vi "EAGLE GUI V5.vi"(9 "TableIn":string[][](table)) -> ()   [LabVIEW 2015]
uses:
  Stream/Controls/RT Status Refs.ctl
  Stream/Robo Team Engine Command.ctl
  Stream/Robo Team Globals.vi
panel:
  out "ViewFinder Sign":picture
  out "Frame Rec":u32
  out "AlgoTime":u32
  out "FrameRate":dbl format="%#.1f"
  out "Stopped":bool
  out "Table Control":string[][](table)
  in  "Ranging":u32
  in  "Aiming":u32
  in  "Illume":u32
  in  "close":bool
  in  "Previous":bool
  in  "Next":bool
  in  "RangingIntensity":u32(slide)=1 caption="Ranging\nIntensity" max=10 step=1 scale=0.0..10.0
  in  "AimingIntensity":u32(slide)=1 caption="Aiming\nIntensity" max=10 step=1 scale=0.0..10.0
  in  "IlluminationIntensity":u32(slide)=1 caption="Illumination\nIntensity" max=10 step=1 scale=0.0..10.0
  out "Iris Found Status":bool
  in  "Tab":enum32{"Page 1", "Page 2", "Page 3"}(tab)
  out "Image":T1(plugin-control)
  # "Treatment Info"
  # "Treatment Process"
  # "Illumination Settings"
  # "Instructions"
  # "1. Adjust illumination\n2. Align the green cross to \n    the center of the pupil\n3. Form cross from the two\n    red lines (Ranging Beams)"
  # "Instructions"
  # "Limbus Border Found\nReady\nClick START"
  # "Instructions"
  # "READY!\n\nClick Start"
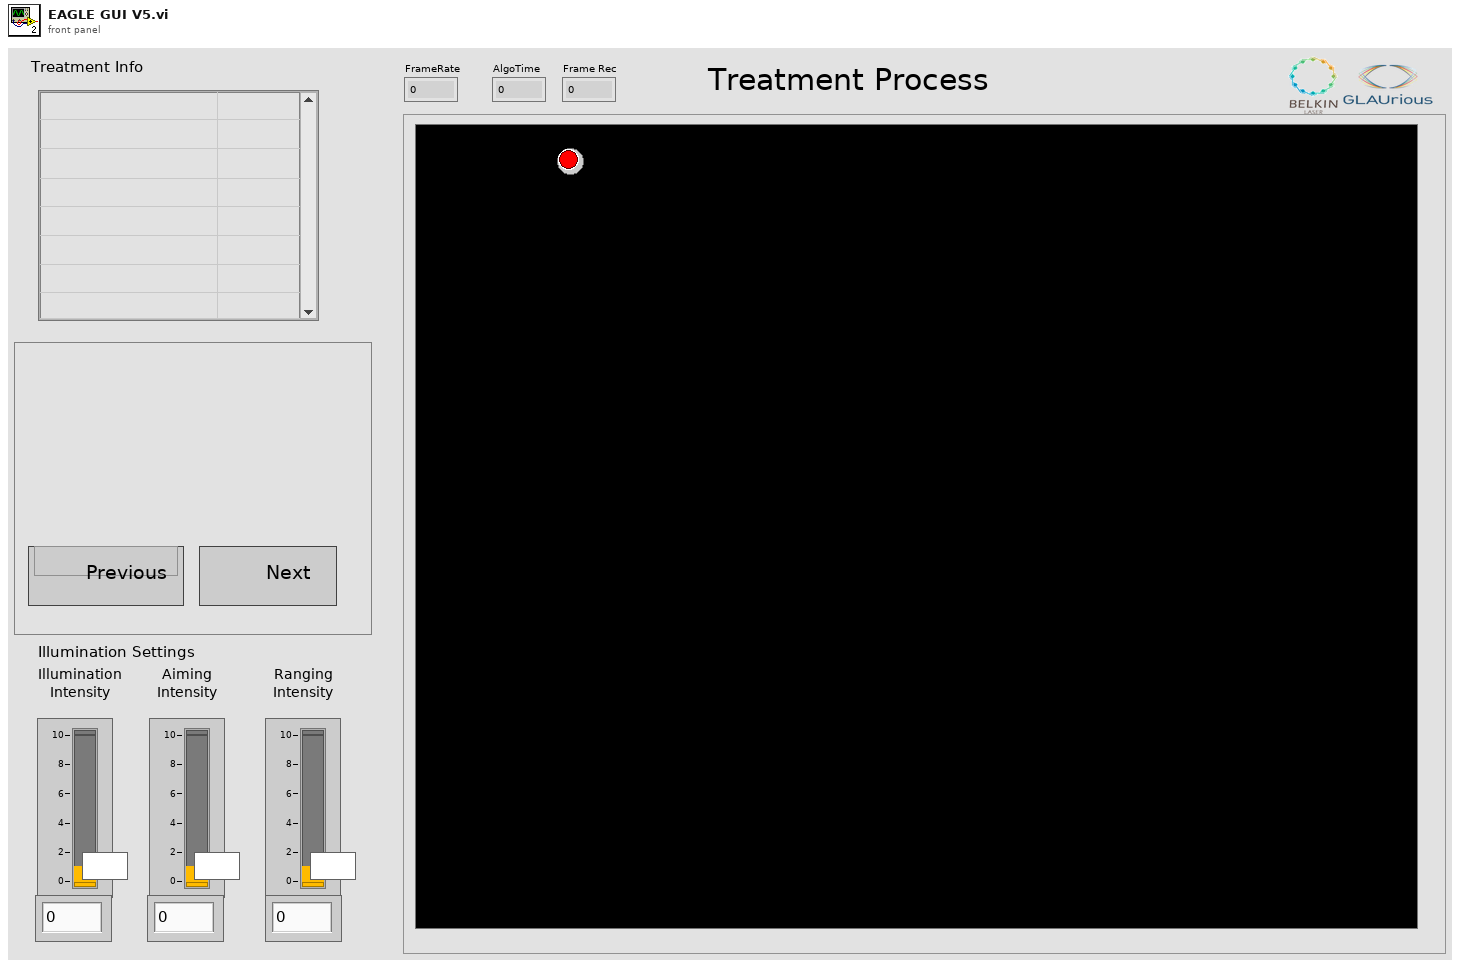
[diagram p1: front panel]
types:
  T1 = typedef "IMAQ Image.ctl" = refnum<image>
  T2 = typedef "RT Status Refs.ctl" = cluster{"Algo Time ref":refnum<vi>, "FrameRate ref":refnum<vi>, "FrameRecRef":refnum<vi>}
  T3 = typedef "Robo Team Engine Command.ctl" = cluster{"Command":string, "Data":variant, "Error":errorcluster, "Timeout":i32}
  T4 = enum8{"Enabled", "Disabled", "Disabled and Grayed Out"}
  T5 = typedef "LVPositionTypeDef.ctl" = cluster{"Left":i32, "Top":i32}
  T6 = typedef "LVRectTypeDef.ctl" = cluster{"Left":i16, "Top":i16, "Right":i16, "Bottom":i16}
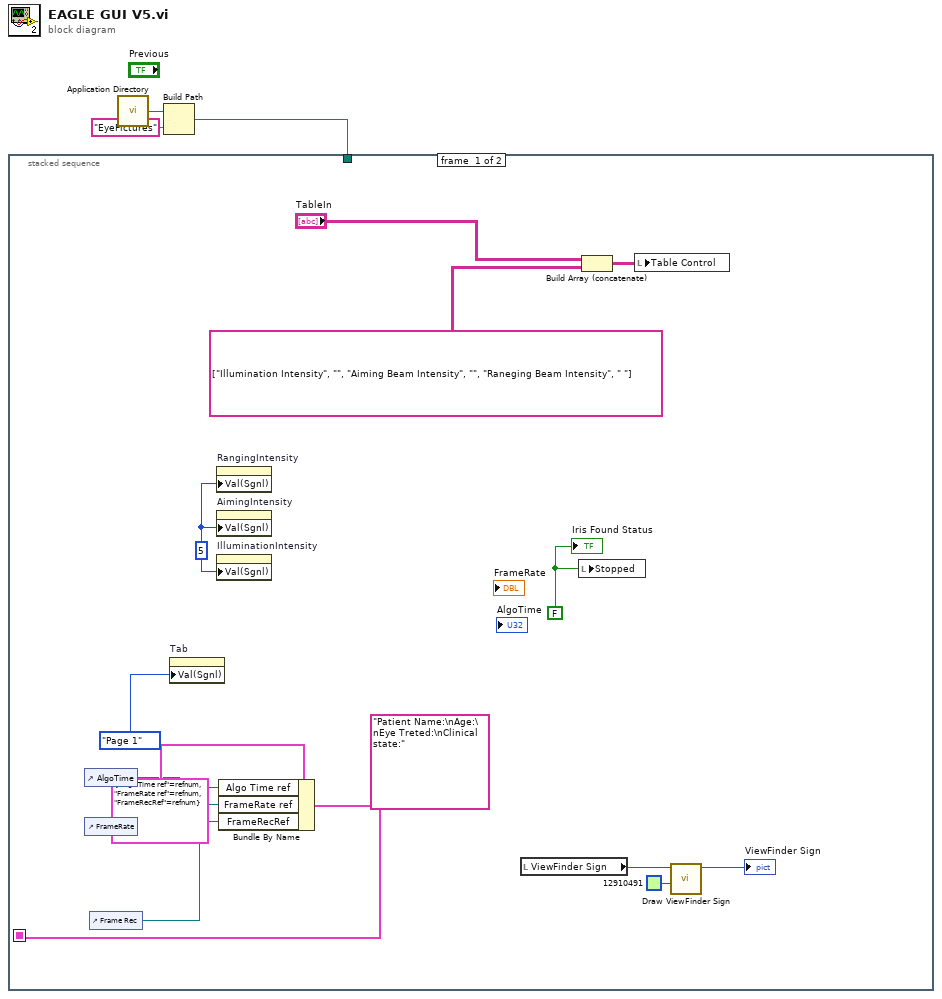
[diagram p0: block diagram]
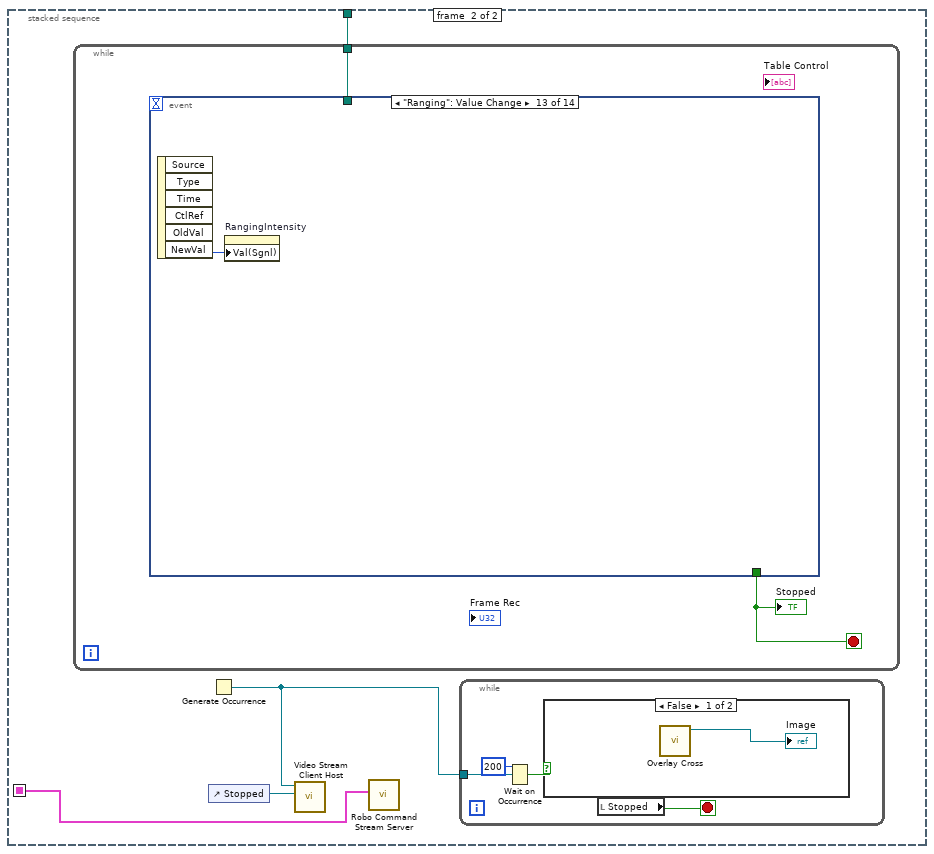
[diagram p2: hidden frame]
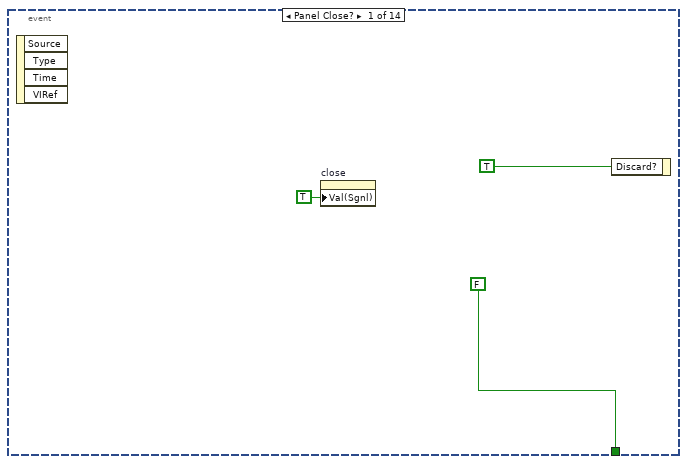
[diagram p4: hidden frame]
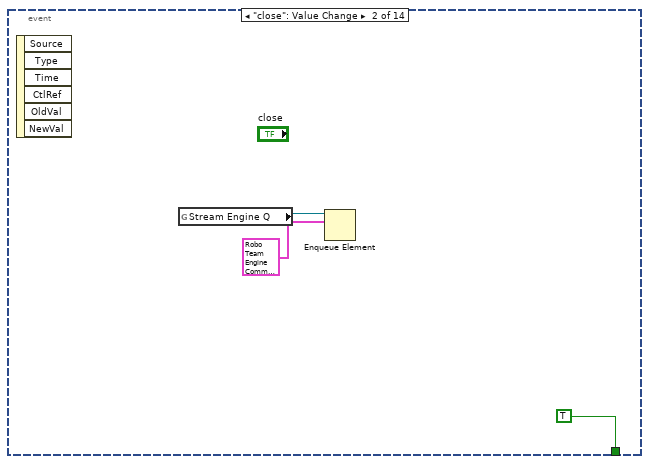
[diagram p5: hidden frame]
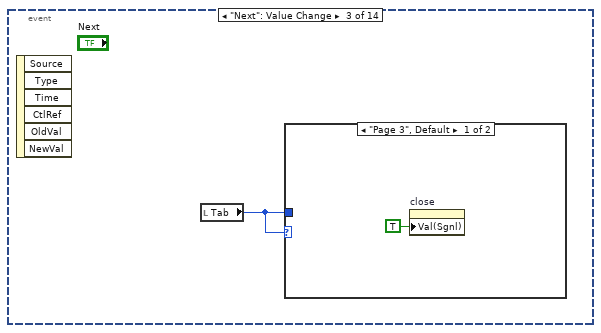
[diagram p6: hidden frame]
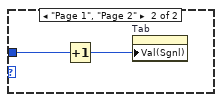
[diagram p7: hidden frame]
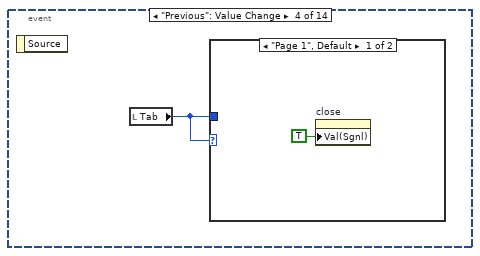
[diagram p8: hidden frame]
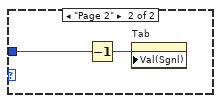
[diagram p9: hidden frame]
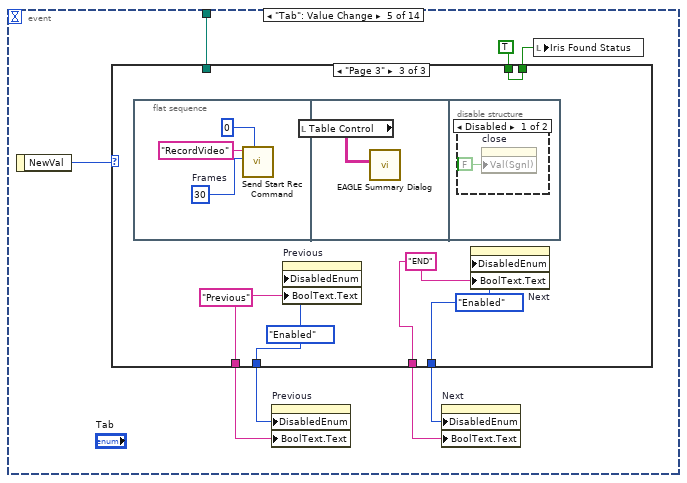
[diagram p10: hidden frame]
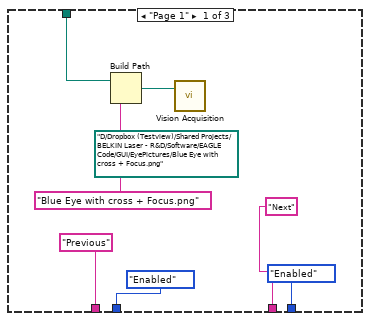
[diagram p11: hidden frame]
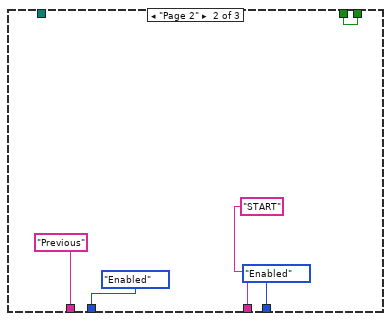
[diagram p12: hidden frame]
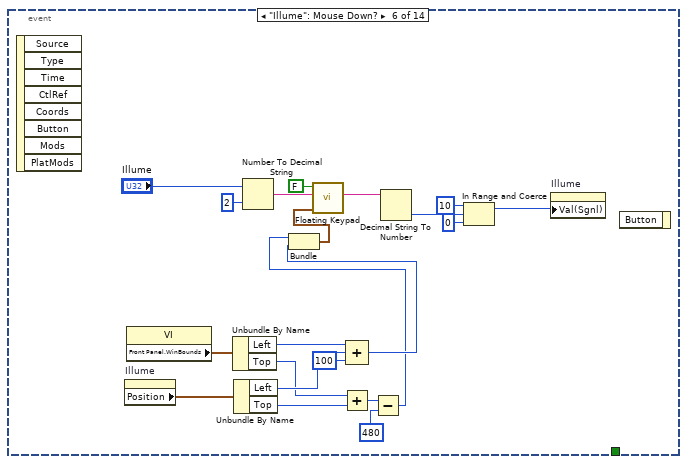
[diagram p14: hidden frame]
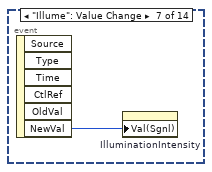
[diagram p15: hidden frame]
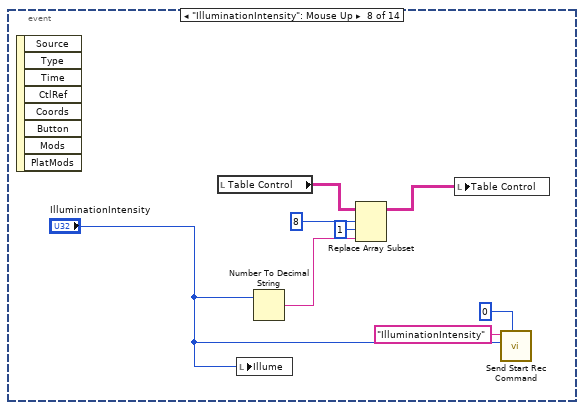
[diagram p16: hidden frame]
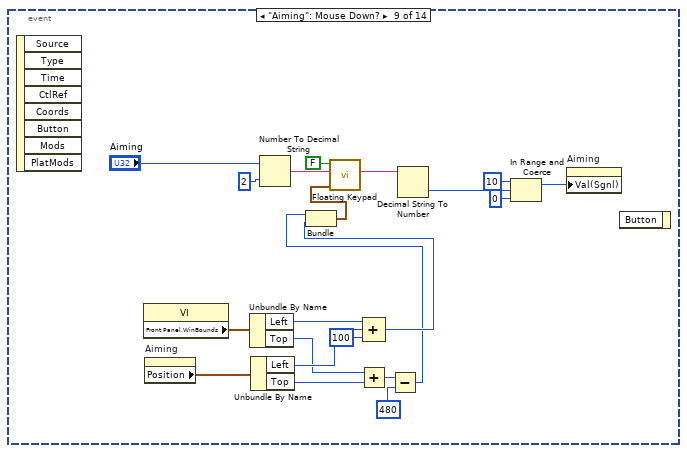
[diagram p17: hidden frame]
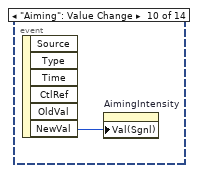
[diagram p18: hidden frame]
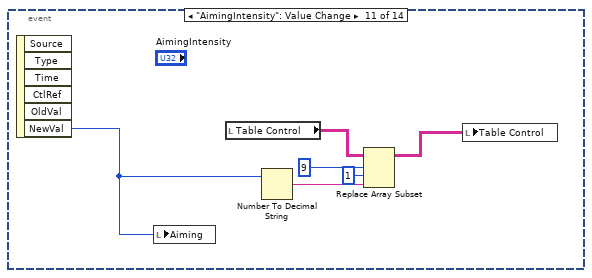
[diagram p19: hidden frame]
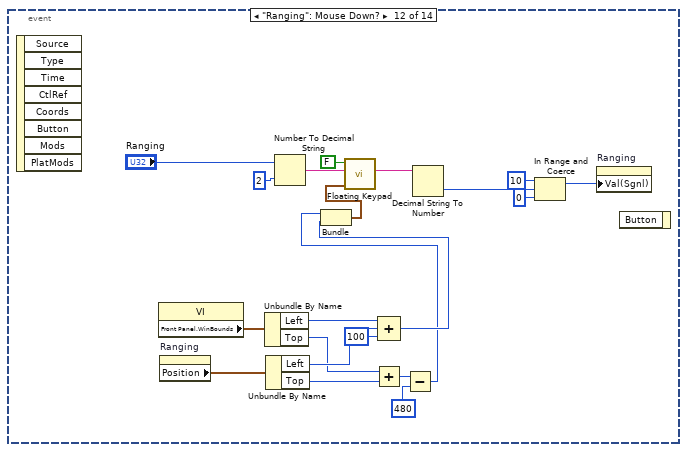
[diagram p20: hidden frame]
diagram:
  n1 = call <vilib>:"Application Directory.vi"() -> ("Application Directory"=w3:path)
  n2 = Build Path(base path=w3, name or relative path="EyePictures") -> (appended path=w1:path)
  n3 = stacked-sequence {
    seq-local: [w10 _] -> [_ w18]
    tunnel: w1 -> [_ w21]
    frame #0 {
      w14 = u32 5 ("Value (Signaling)")
      w12 = FALSE ("Iris Found Status")
      (unwired) "Patient Name:\nAge:\nEye Treted:\nClinical state:" ("patient Info")
      n4 = control-ref of="AlgoTime"() -> (w8:refnum<vi>)
      n5 = control-ref of="FrameRate"() -> (w9:refnum<vi>)
      n6 = control-ref of="Frame Rec"() -> (w7:refnum<vi>)
      n7 = property on="Tab" class="TabCtl (strict)"("Val(Sgnl)"=enum32{"Page 1", "Page 2"}."Page 1" ("Tab")) -> ()  [unwired: 2 in, 2 out]
      n8 = property on="RangingIntensity" class="Slide (strict)"("Val(Sgnl)"=w14) -> ()  [unwired: 2 in, 2 out]
      n9 = property on="AimingIntensity" class="Slide (strict)"("Val(Sgnl)"=w14) -> ()  [unwired: 2 in, 2 out]
      n10 = property on="IlluminationIntensity" class="Slide (strict)"("Val(Sgnl)"=w14) -> ()  [unwired: 2 in, 2 out]
      n11 = Bundle By Name(cluster=T2 {"Algo Time ref"=refnum, "FrameRate ref"=refnum, "FrameRecRef"=refnum} ("StatusRefs"), "Algo Time ref"=w8, "FrameRate ref"=w9, "FrameRecRef"=w7) -> (w10:T2)
      n12 = local read "ViewFinder Sign"() -> (w6:picture)
      n13 = local write "Stopped"(w12) -> ()
      n14 = Build Array (concatenate)("TableIn", string[][] [["Illumination Intensity", ""], ["Aiming Beam Intensity", ""], ["Raneging Beam Intensity", " "]] ("Table Control")) -> (w13:string[][])
      n15 = local write "Table Control"(w13) -> ()
      n16 = call "Draw ViewFinder Sign.vi"("Color"=u32 12910491, "2D Picture"=w6) -> ("2D Picture out"=→"ViewFinder Sign":picture)  [unwired: 9 in]
      "Iris Found Status" <- w12
    }
    frame #1 {
      n17 = while {
        tunnel: w21 -> [w27]
        stop <- w28 stop-if-true
        n18 = event shown="[12] \"Ranging\": Value Change" {
          selector: _ -> [_ _ _ _ _ _ _ _ _ _ _ _ _ _]
          dyn-events: _ -> [_ _ _ _ _ _ _ _ _ _ _ _ _ _]
          timeout: _ -> [_ _ _ _ _ _ _ _ _ _ _ _ _ _]
          tunnel: [FALSE TRUE _ _ _ _ _ _ _ _ _ _ _ _] -> w28
          tunnel: w27 -> [_ _ _ _ w43 _ _ _ _ _ _ _ _ _]
          event Panel Close? {
            n19 = event-data() -> ()  [unwired: 1 in, 4 out]
            n20 = property on="close" class="Bool (strict)"("Val(Sgnl)"=TRUE ("Value (Signaling)")) -> ()  [unwired: 2 in, 2 out]
            n21 = event-data("Discard?"=TRUE) -> ()  [unwired: 1 in, 1 out]
          }
          event "close": Value Change {
            n22 = event-data() -> ()  [unwired: 1 in, 6 out]
            n23 = global read "Robo Team Globals.vi" "Stream Engine Q"() -> (w33:refnum<queue>)
            n24 = Enqueue Element(queue=w33, element=T3 {"Command"="Close", "Data"=variant, "Error"={"status"=FALSE, "code"=0, "source"=""}, "Timeout"=0}) -> ()  [unwired: 2 in, 3 out]
          }
          event "Next": Value Change {
            n25 = event-data() -> ()  [unwired: 1 in, 6 out]
            n26 = local read "Tab"() -> (w35:enum32{"Page 1", "Page 2", "Page 3"})
            n27 = case shown="\"Page 3\", Default" w35 {
              tunnel: w35 -> [_ w37]
              frame "Page 3", Default {
                n28 = property on="close" class="Bool (strict)"("Val(Sgnl)"=TRUE ("Value (Signaling)")) -> ()  [unwired: 2 in, 2 out]
              }
              frame "Page 1", "Page 2" {
                n29 = Increment(x=w37) -> (x+1=w38:enum32{"Page 1", "Page 2", "Page 3"})
                n30 = property on="Tab" class="TabCtl (strict)"("Val(Sgnl)"=w38) -> ()  [unwired: 2 in, 2 out]
              }
            }
          }
          event "Previous": Value Change {
            n31 = event-data() -> ()  [unwired: 1 in, 1 out]
            n32 = local read "Tab"() -> (w39:enum32{"Page 1", "Page 2", "Page 3"})
            n33 = case shown="\"Page 1\", Default" w39 {
              tunnel: w39 -> [_ w42]
              frame "Page 1", Default {
                n34 = property on="close" class="Bool (strict)"("Val(Sgnl)"=TRUE ("Value (Signaling)")) -> ()  [unwired: 2 in, 2 out]
              }
              frame "Page 2" {
                n35 = Decrement(x=w42) -> (x-1=w41:enum32{"Page 1", "Page 2", "Page 3"})
                n36 = property on="Tab" class="TabCtl (strict)"("Val(Sgnl)"=w41) -> ()  [unwired: 2 in, 2 out]
              }
            }
          }
          event "Tab": Value Change {
            n37 = event-data() -> ("NewVal"=w50:enum32{"Page 1", "Page 2", "Page 3"})  [unwired: 1 in]
            n38 = case shown="\"Page 3\"" w50 {
              tunnel: [T4."Enabled" ("Disabled") T4."Enabled" ("Disabled") w63] -> w49
              tunnel: [T4."Enabled" ("Disabled") T4."Enabled" ("Disabled") w65] -> w48
              tunnel: ["Next" "START" w66] -> w47
              tunnel: ["Previous" "Previous" w64] -> w46
              tunnel: [_ w58 w67] -> w45
              tunnel: TRUE -> [_ w58 w67]
              tunnel: w43 -> [w53 _ _]
              frame "Page 1" {
                (unwired) path "D:/Dropbox (Testview)/Shared Projects/BELKIN Laser - R&D/Software/EAGLE Code/GUI/EyePictures/Blue Eye with cross + Focus.png" ("Image Path")
                n39 = Build Path(base path=w53, name or relative path="Blue Eye with cross + Focus.png") -> (appended path=w51:path)
                n40 = call "Vision Acquisition"("Image Path"=w51) -> ()  [unwired: 25 in, 2 out]
              }
              frame "Page 2" {
              }
              frame "Page 3" {
                w64 = "Previous"
                w66 = "END"
                w63 = T4."Enabled" ("Disabled")
                w65 = T4."Enabled" ("Disabled")
                n41 = flat-sequence {
                  frame #0 {
                    w69 = 30  # Frames
                    n42 = call "Send Start Rec Command.vi"("timeout in ms (5000)"=0, "Data in"=w69, "Command"="RecordVideo") -> ()  [unwired: 7 in, 2 out]
                  }
                  frame #1 {
                    n43 = local read "Table Control"() -> (w71:string[][])
                    n44 = call "EAGLE Summary Dialog.vi"("Table Control in"=w71) -> ()  [unwired: 11 in]
                  }
                  frame #2 {
                    n45 = disable-structure shown="Disabled" {
                      frame Disabled {
                        n46 = property on="close" class="Bool (strict)"("Val(Sgnl)"=FALSE ("Value (Signaling)")) -> ()  [unwired: 2 in, 2 out]
                      }
                      frame Enabled {
                      }
                    }
                  }
                }
                n47 = property on="Previous" class="Bool"("DisabledEnum"=w63, "BoolText.Text"=w64) -> ()  [unwired: 2 in, 2 out]
                n48 = property on="Next" class="Bool"("DisabledEnum"=w65, "BoolText.Text"=w66) -> ()  [unwired: 2 in, 2 out]
              }
            }
            n49 = property on="Previous" class="Bool"("DisabledEnum"=w49, "BoolText.Text"=w46) -> ()  [unwired: 2 in, 2 out]
            n50 = property on="Next" class="Bool"("DisabledEnum"=w48, "BoolText.Text"=w47) -> ()  [unwired: 2 in, 2 out]
            n51 = local write "Iris Found Status"(w45) -> ()
          }
          event "Illume": Mouse Down? {
            n52 = event-data() -> ()  [unwired: 1 in, 8 out]
            n53 = property on="Illume" class="DigNum (strict)"() -> ("Position"=w78:T5)  [unwired: 2 in, 2 out]
            n54 = property class="VI"() -> ("Front Panel.WinBounds"=w77:T6)  [unwired: 2 in, 2 out]
            n55 = Unbundle By Name(w77) -> ("Left"=w90:i16, "Top"=w87:i16)
            n56 = Unbundle By Name(w78) -> ("Left"=w89:i32, "Top"=w88:i32)
            n57 = Number To Decimal String(number="Illume", width (-)=i16 2 ("precision (6)")) -> (decimal integer string=w93:string)
            n58 = Add(x=w87, y=w88) -> (x+y=w84:i32)
            n59 = Compound Arithmetic op=ADD(w90, w89, 100 ("value")) -> (w85:i32)
            n60 = Subtract(x=w84, y=480) -> (x-y=w82:i32)
            n61 = Bundle(w82, w85) -> (w81:cluster{i32, i32})  [unwired: 1 in]
            n62 = call "Floating Keypad.vi"("Position"=w81, "StringIn"=w93, "Allow dot"=FALSE) -> ("StringOut"=w92:string)  [unwired: 8 in]
            n63 = Decimal String To Number(string=w92) -> (number=w76:i32)  [unwired: 2 in, 1 out]
            n64 = In Range and Coerce(upper limit=10, x=w76, lower limit=0) -> (coerced(x)=w75:i32)  [unwired: 1 out]
            n65 = property on="Illume" class="DigNum (strict)"("Val(Sgnl)"=w75) -> ()  [unwired: 2 in, 2 out]
            n66 = event-data() -> ()  [unwired: 2 in, 1 out]
          }
          event "Illume": Value Change {
            n67 = event-data() -> ("NewVal"=w94:u32)  [unwired: 1 in, 5 out]
            n68 = property on="IlluminationIntensity" class="Slide (strict)"("Val(Sgnl)"=w94) -> ()  [unwired: 2 in, 2 out]
          }
          event "IlluminationIntensity": Mouse Up {
            n69 = event-data() -> ()  [unwired: 1 in, 8 out]
            n70 = local read "Table Control"() -> (w102:string[][])
            n71 = local write "Illume"("IlluminationIntensity") -> ()
            n72 = Number To Decimal String(number="IlluminationIntensity") -> (decimal integer string=w98:string)  [unwired: 1 in]
            n73 = Replace Array Subset(array=w102, new element=w98, index (row)=8 ("disabled index (row)"), index (col)=1 ("disabled index (col)")) -> (w101:string[][])
            n74 = local write "Table Control"(w101) -> ()
            n75 = call "Send Start Rec Command.vi"("timeout in ms (5000)"=0, "Data in"="IlluminationIntensity", "Command"="IlluminationIntensity") -> ()  [unwired: 7 in, 2 out]
          }
          event "Aiming": Mouse Down? {
            n76 = event-data() -> ()  [unwired: 1 in, 8 out]
            n77 = property class="VI"() -> ("Front Panel.WinBounds"=w107:T6)  [unwired: 2 in, 2 out]
            n78 = property on="Aiming" class="DigNum (strict)"() -> ("Position"=w108:T5)  [unwired: 2 in, 2 out]
            n79 = Unbundle By Name(w107) -> ("Left"=w120:i16, "Top"=w117:i16)
            n80 = Unbundle By Name(w108) -> ("Left"=w119:i32, "Top"=w118:i32)
            n81 = Number To Decimal String(number="Aiming", width (-)=i16 2 ("precision (6)")) -> (decimal integer string=w123:string)
            n82 = Add(x=w117, y=w118) -> (x+y=w114:i32)
            n83 = Compound Arithmetic op=ADD(w120, w119, 100 ("value")) -> (w115:i32)
            n84 = Subtract(x=w114, y=480) -> (x-y=w112:i32)
            n85 = Bundle(w112, w115) -> (w111:cluster{i32, i32})  [unwired: 1 in]
            n86 = call "Floating Keypad.vi"("Position"=w111, "StringIn"=w123, "Allow dot"=FALSE) -> ("StringOut"=w122:string)  [unwired: 8 in]
            n87 = Decimal String To Number(string=w122) -> (number=w104:i32)  [unwired: 2 in, 1 out]
            n88 = In Range and Coerce(upper limit=10, x=w104, lower limit=0) -> (coerced(x)=w103:i32)  [unwired: 1 out]
            n89 = property on="Aiming" class="DigNum (strict)"("Val(Sgnl)"=w103) -> ()  [unwired: 2 in, 2 out]
            n90 = event-data() -> ()  [unwired: 2 in, 1 out]
          }
          event "Aiming": Value Change {
            n91 = event-data() -> ("NewVal"=w124:u32)  [unwired: 1 in, 5 out]
            n92 = property on="AimingIntensity" class="Slide (strict)"("Val(Sgnl)"=w124) -> ()  [unwired: 2 in, 2 out]
          }
          event "AimingIntensity": Value Change {
            n93 = event-data() -> ("NewVal"=w125:u32)  [unwired: 1 in, 5 out]
            n94 = local write "Aiming"(w125) -> ()
            n95 = local read "Table Control"() -> (w130:string[][])
            n96 = Number To Decimal String(number=w125) -> (decimal integer string=w126:string)  [unwired: 1 in]
            n97 = Replace Array Subset(array=w130, new element=w126, index (row)=9 ("disabled index (row)"), index (col)=1 ("disabled index (col)")) -> (w129:string[][])
            n98 = local write "Table Control"(w129) -> ()
          }
          event "Ranging": Mouse Down? {
            n99 = event-data() -> ()  [unwired: 1 in, 8 out]
            n100 = property class="VI"() -> ("Front Panel.WinBounds"=w135:T6)  [unwired: 2 in, 2 out]
            n101 = property on="Ranging" class="DigNum (strict)"() -> ("Position"=w136:T5)  [unwired: 2 in, 2 out]
            n102 = Unbundle By Name(w135) -> ("Left"=w148:i16, "Top"=w145:i16)
            n103 = Unbundle By Name(w136) -> ("Left"=w147:i32, "Top"=w146:i32)
            n104 = Number To Decimal String(number="Ranging", width (-)=i16 2 ("precision (6)")) -> (decimal integer string=w151:string)
            n105 = Add(x=w145, y=w146) -> (x+y=w142:i32)
            n106 = Compound Arithmetic op=ADD(w148, w147, 100 ("value")) -> (w143:i32)
            n107 = Subtract(x=w142, y=480) -> (x-y=w140:i32)
            n108 = Bundle(w140, w143) -> (w139:cluster{i32, i32})  [unwired: 1 in]
            n109 = call "Floating Keypad.vi"("Position"=w139, "StringIn"=w151, "Allow dot"=FALSE) -> ("StringOut"=w150:string)  [unwired: 8 in]
            n110 = Decimal String To Number(string=w150) -> (number=w132:i32)  [unwired: 2 in, 1 out]
            n111 = In Range and Coerce(upper limit=10, x=w132, lower limit=0) -> (coerced(x)=w131:i32)  [unwired: 1 out]
            n112 = property on="Ranging" class="DigNum (strict)"("Val(Sgnl)"=w131) -> ()  [unwired: 2 in, 2 out]
            n113 = event-data() -> ()  [unwired: 2 in, 1 out]
          }
          event "Ranging": Value Change {
            n114 = event-data() -> ("NewVal"=w152:u32)  [unwired: 1 in, 5 out]
            n115 = property on="RangingIntensity" class="Slide (strict)"("Val(Sgnl)"=w152) -> ()  [unwired: 2 in, 2 out]
          }
          event "RangingIntensity": Value Change {
            n116 = event-data() -> ()  [unwired: 1 in, 6 out]
            n117 = local write "Ranging"("RangingIntensity") -> ()
            n118 = local read "Table Control"() -> (w158:string[][])
            n119 = Number To Decimal String(number="RangingIntensity") -> (decimal integer string=w154:string)  [unwired: 1 in]
            n120 = Replace Array Subset(array=w158, new element=w154, index (row)=10 ("disabled index (row)"), index (col)=1 ("disabled index (col)")) -> (w157:string[][])
            n121 = local write "Table Control"(w157) -> ()
          }
        }
        "Stopped" <- w28
      }
      n122 = Generate Occurrence() -> (w19:refnum<k4>)
      n123 = control-ref of="Stopped"() -> (w20:refnum<vi>)
      n124 = call "Video Stream Client Host.vi"("Close ref"=w20, "occurrence"=w19) -> ()  [unwired: 10 in]
      n125 = call "Robo Command Stream Server.vi"("StatusRefs"=w18) -> ()  [unwired: 11 in]
      n126 = while {
        tunnel: w19 -> [w24]
        stop <- w25 stop-if-true
        n127 = Wait on Occurrence(2:w24, 3:200 ("ms timeout (-1)")) -> (0:w22:bool)  [unwired: 1 in]
        n128 = case shown="False" w22 {
          frame False {
            n129 = call "Overlay Cross.vi"() -> ("Image Out"=→"Image":T1)  [unwired: 11 in]
          }
          frame True {
          }
        }
        n130 = local read "Stopped"() -> (w25:bool)
      }
    }
  }
